vi "Tellegen's Theorem_26_08_2014.vi"() -> ()   [LabVIEW 2011]
panel:
  out "Switch 4":bool
  out "Ammeter 3":dbl(knob) scale=-5.0..5.0
  out "Switch":bool
  out "Ammeter 2":dbl(knob) scale=-5.0..5.0
  out "Switch":bool
  out "Ammeter":dbl(knob) scale=-5.0..5.0 scale format="%#.6g"
  in  "Circuit Select":enum32{"Case1 ", "Case 2", "Case 3"}(tab)
  out "Table-1(Case-1)":string[][](table)
  out "Table 2(Case-2)":string[][](table)
  out "Table 3 (case-3)":string[][](table)
  in  "Voltage(V2)":dbl
  in  "Voltage(V1)":dbl
  in  "R3":dbl=29.3001 min=1e-05 max=50.0 step=0.05
  in  "R2":dbl=119.7 min=1e-06 max=185.0 step=0.05
  in  "R1":dbl=49.8001 min=1e-05 max=85.0 step=0.05
  in  "S1(DPDT)":enum16{"POWER", "SHORT"}(ring)
  in  "S2(DPDT)":enum16{"POWER", "SHORT"}(ring)
  out "Switch 2":bool
  out "Switch 1":bool
  # "Tellegen's  Theorem"
  # "Experiment Part Select        \nSet all the resistance R1, R2, R3 and set the voltages V1 and V2.       \n   \nCase-1: Select switch of S1 and S2 . Simulate the program . Observe the result from Case 1.\n    \n Case-2: \n a) Apply switch S1 to \"Power\" and S2 to \"Short\". Simulate the program.\nObserve the all branches current  and branch volatge from Case 2 tab.\n\n \nCase-3: a) Apply switch S1 to \"Short\" and S2 to \"Power\". Simulate the program.\nObserve the all branches current  and branch volatge from Case 2 tab.\n\n\n \n    \n       MC-Moving Coil.\n       DPDT- Double pole Double throw."
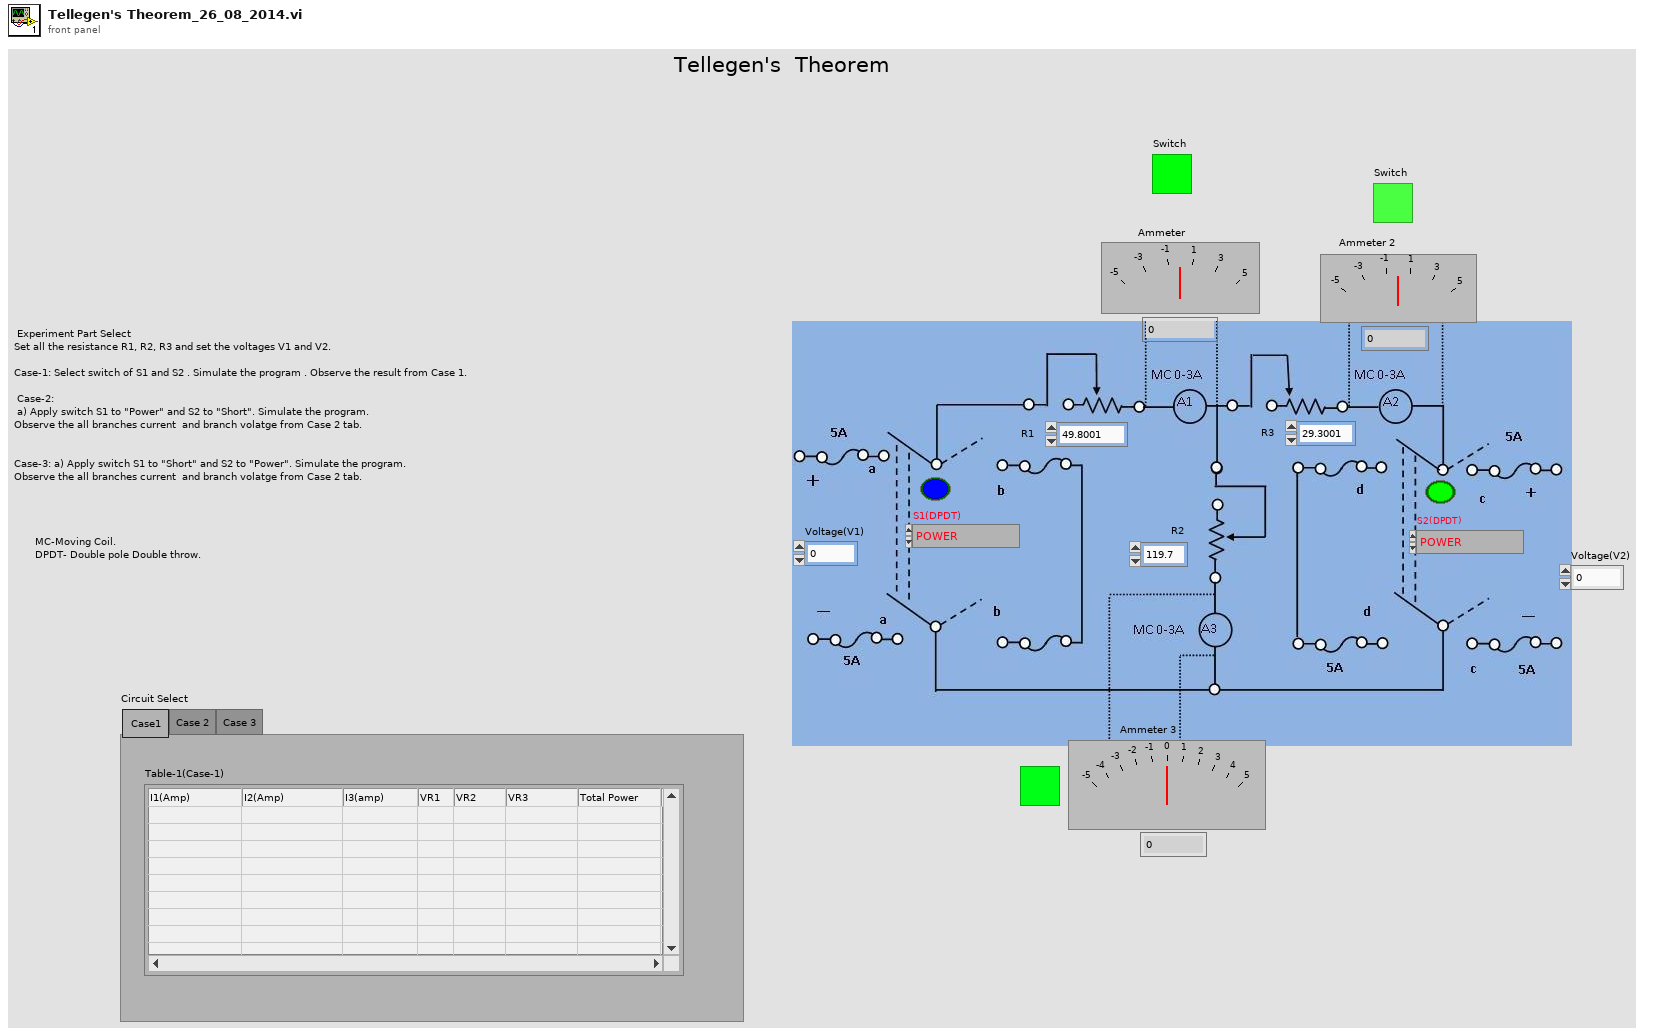
[diagram p1: front panel]
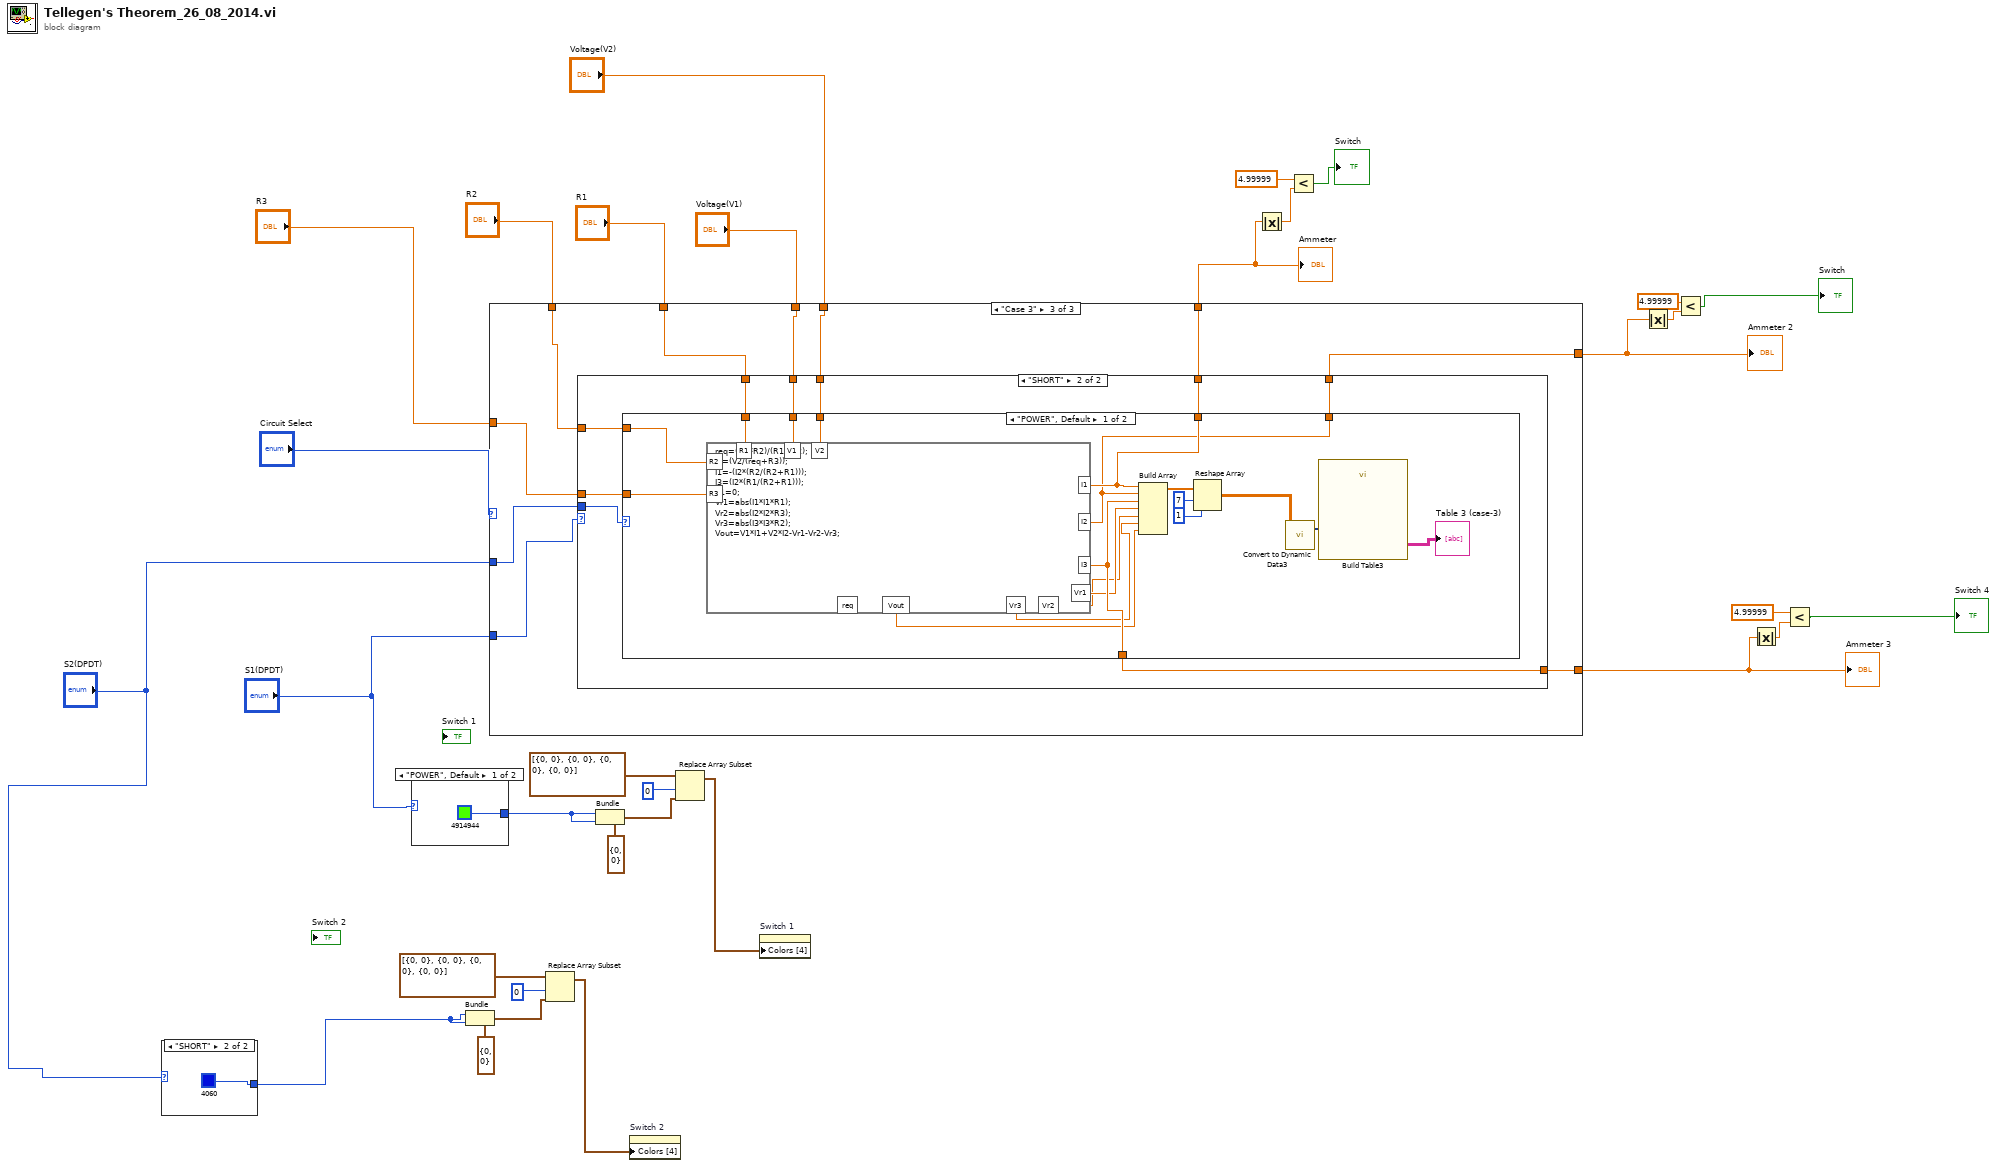
[diagram p0: block diagram]
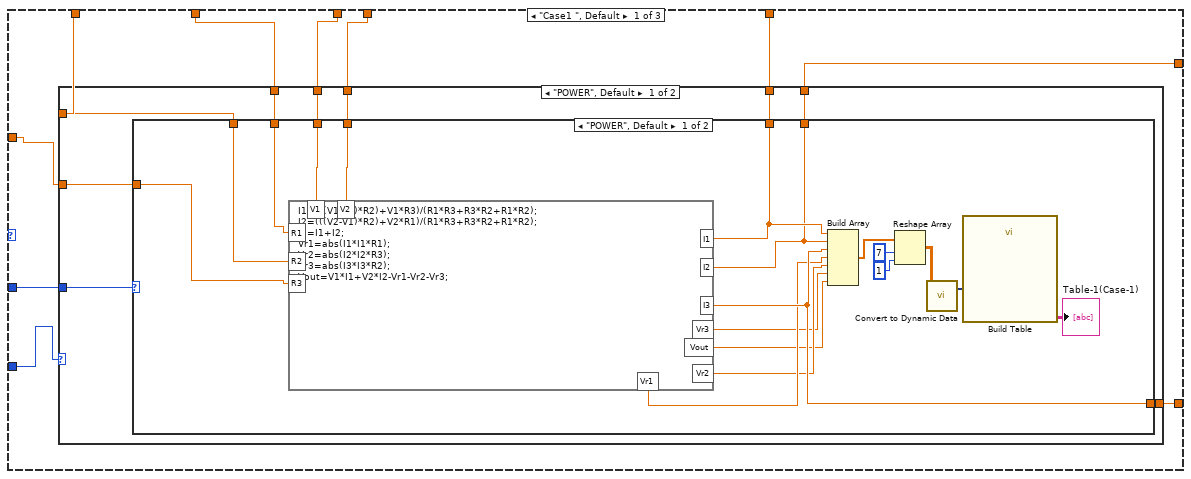
[diagram p2: hidden frame]
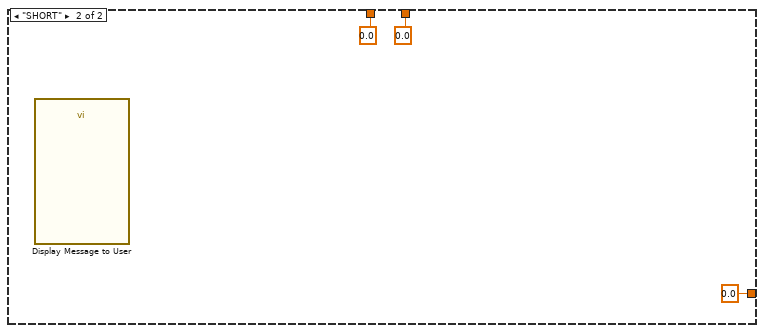
[diagram p3: hidden frame]
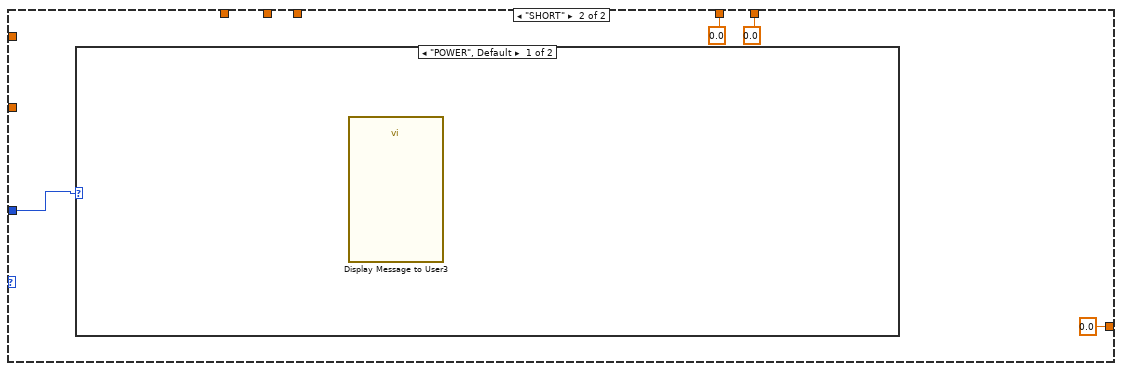
[diagram p4: hidden frame]
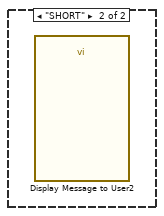
[diagram p5: hidden frame]
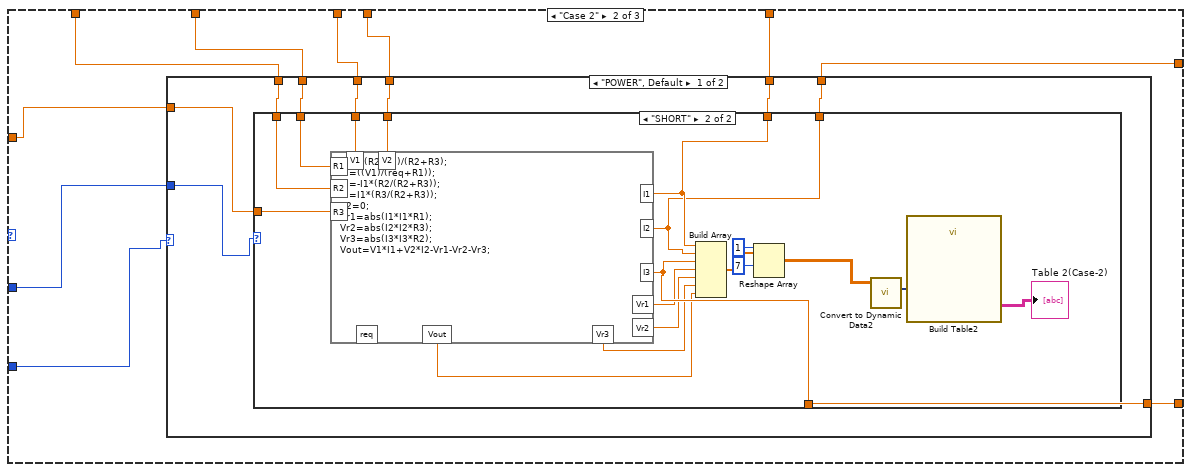
[diagram p6: hidden frame]
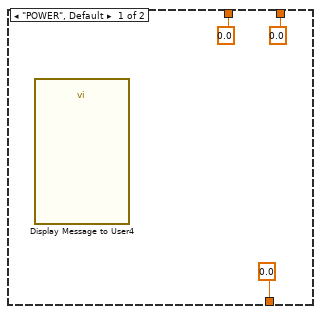
[diagram p7: hidden frame]
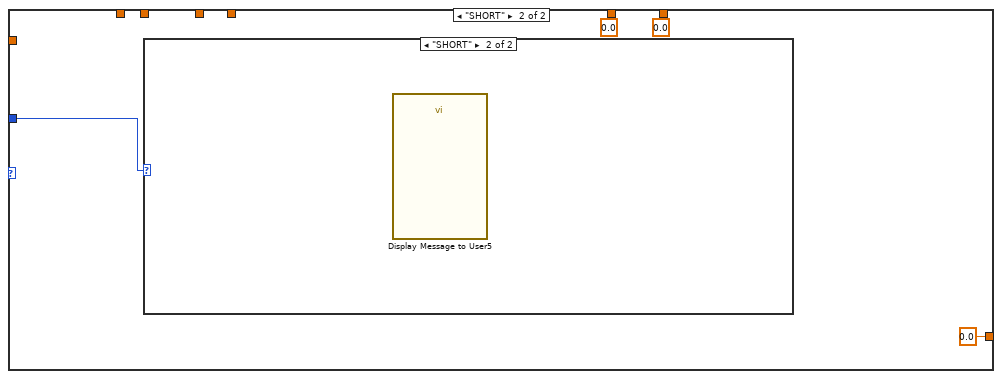
[diagram p8: hidden frame]
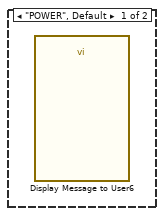
[diagram p9: hidden frame]
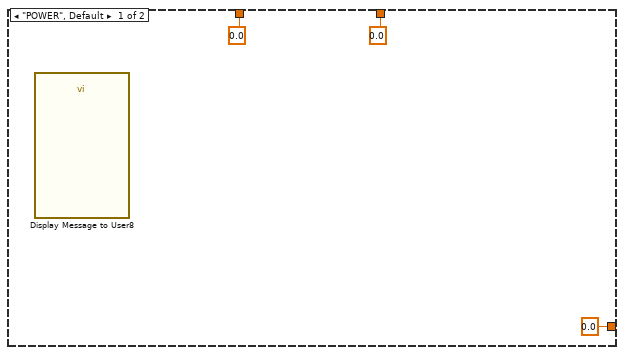
[diagram p10: hidden frame]
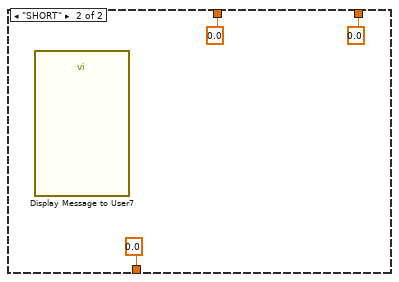
[diagram p11: hidden frame]
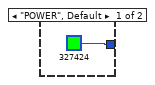
[diagram p12: hidden frame]
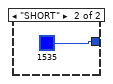
[diagram p13: hidden frame]
diagram:
  n1 = case shown="\"SHORT\"" "S2(DPDT)" {
    tunnel: [u32 327424 u32 4060] -> w21
    frame "POWER", Default {
    }
    frame "SHORT" {
    }
  }
  n2 = case shown="\"POWER\", Default" "S1(DPDT)" {
    tunnel: [u32 4914944 u32 1535] -> w28
    frame "POWER", Default {
    }
    frame "SHORT" {
    }
  }
  n3 = Bundle(cluster=cluster{u32, u32} {0, 0}, w21, w21) -> (w24:cluster{u32, u32})
  n4 = case shown="\"Case 3\"" "Circuit Select" {
    tunnel: "S1(DPDT)" -> [w41 w90 w134]
    tunnel: "Voltage(V1)" -> [w45 w87 w129]
    tunnel: "Voltage(V2)" -> [w46 w88 w128]
    tunnel: "R1" -> [w44 w86 w132]
    tunnel: "R2" -> [w43 w85 w131]
    tunnel: "R3" -> [w42 w84 w130]
    tunnel: "S2(DPDT)" -> [w40 w89 w133]
    tunnel: [w39 w83 w127] -> w9
    tunnel: [w38 w82 w126] -> w1
    tunnel: [w37 w81 w125] -> w2
    frame "Case1 ", Default {
      n5 = case shown="\"POWER\", Default" w41 {
        tunnel: w45 -> [w55 _]
        tunnel: w44 -> [w54 _]
        tunnel: w42 -> [w53 _]
        tunnel: w46 -> [w52 _]
        tunnel: w43 -> [w51 _]
        tunnel: w40 -> [w50 w80]
        tunnel: [w49 0.0 ("I1")] -> w39
        tunnel: [w48 0.0 ("I2")] -> w38
        tunnel: [w47 0.0 ("I3")] -> w37
        frame "POWER", Default {
          n6 = case shown="\"POWER\", Default" w50 {
            tunnel: w52 -> [w73 _]
            tunnel: w55 -> [w72 _]
            tunnel: w54 -> [w71 _]
            tunnel: w51 -> [w70 _]
            tunnel: w53 -> [w69 _]
            tunnel: [w62 0.0 ("I1")] -> w49
            tunnel: [w61 0.0 ("I2")] -> w48
            tunnel: [w60 0.0 ("I3")] -> w47
            frame "POWER", Default {
              n7 = formula code="I1=(((V1-V2)*R2)+V1*R3)/(R1*R3+R3*R2+R1*R2);\nI2=(((V2-V1)*R2)+V2*R1)/(R1*R3+R3*R2+R1*R2);\nI3=I1+I2;\nVr1=abs(I1*I1*R1);\nVr2=abs(I2*I2*R3);\nVr3=abs(I3*I3*R2);\nVout=V1*I1+V2*I2-Vr1-Vr2-Vr3;"("V1"=w72, "V2"=w73, "R1"=w71, "R2"=w70, "R3"=w69) -> ("I1"=w62:dbl, "I2"=w61:dbl, "I3"=w60:dbl, "Vout"=w56:dbl, "Vr1"=w59:dbl, "Vr3"=w57:dbl, "Vr2"=w58:dbl)
              n8 = Build Array(w62, w61, w60, w59, w58, w57, w56) -> (w67:dbl[])
              n9 = Reshape Array(w67, 7 ("dimension size"), 1 ("dimension size")) -> (w64:dbl[][])
              n10 = call "Convert to Dynamic Data"("2D Array"=w64) -> ("Dynamic Data Type"=w63:dynamicdata)  [unwired: 3 out]
              n11 = call "Build Table"("Signals"=w63) -> ("Table"=→"Table-1(Case-1)":string[][])  [unwired: 4 in, 6 out]
            }
            frame "SHORT" {
              n12 = call "Display Message to User"() -> ()  [unwired: 10 in, 2 out]
            }
          }
        }
        frame "SHORT" {
          n13 = case shown="\"POWER\", Default" w80 {
            frame "POWER", Default {
              n14 = call "Display Message to User3"() -> ()  [unwired: 10 in, 2 out]
            }
            frame "SHORT" {
              n15 = call "Display Message to User2"() -> ()  [unwired: 10 in, 2 out]
            }
          }
        }
      }
    }
    frame "Case 2" {
      n16 = case shown="\"POWER\", Default" w90 {
        tunnel: w89 -> [w99 w124]
        tunnel: w88 -> [w98 _]
        tunnel: w87 -> [w97 _]
        tunnel: w86 -> [w96 _]
        tunnel: w85 -> [w95 _]
        tunnel: w84 -> [w94 _]
        tunnel: [w93 0.0 ("I1")] -> w83
        tunnel: [w92 0.0 ("I2")] -> w82
        tunnel: [w91 0.0 ("I3")] -> w81
        frame "POWER", Default {
          n17 = case shown="\"SHORT\"" w99 {
            tunnel: w98 -> [_ w120]
            tunnel: w97 -> [_ w119]
            tunnel: w96 -> [_ w118]
            tunnel: w95 -> [_ w117]
            tunnel: w94 -> [_ w116]
            tunnel: [0.0 ("I1") w110] -> w93
            tunnel: [0.0 ("I2") w109] -> w92
            tunnel: [0.0 ("I3") w108] -> w91
            frame "POWER", Default {
              n18 = call "Display Message to User4"() -> ()  [unwired: 10 in, 2 out]
            }
            frame "SHORT" {
              n19 = formula code="req=(R2*R3)/(R2+R3);\nI1=((V1)/(req+R1));\nI2=-I1*(R2/(R2+R3));\nI3=I1*(R3/(R2+R3));\nV2=0;\nVr1=abs(I1*I1*R1);\nVr2=abs(I2*I2*R3);\nVr3=abs(I3*I3*R2);\nVout=V1*I1+V2*I2-Vr1-Vr2-Vr3;"("V2"=w120, "V1"=w119, "R1"=w118, "R2"=w117, "R3"=w116) -> ("I1"=w110:dbl, "I2"=w109:dbl, "I3"=w108:dbl, "Vr1"=w107:dbl, "Vr2"=w106:dbl, "Vr3"=w105:dbl, "Vout"=w103:dbl)  [unwired: 1 out]
              n20 = Build Array(w110, w109, w108, w107, w106, w105, w103) -> (w104:dbl[])
              n21 = Reshape Array(w104, 7 ("dimension size"), 1 ("dimension size")) -> (w112:dbl[][])
              n22 = call "Convert to Dynamic Data2"("2D Array"=w112) -> ("Dynamic Data Type"=w111:dynamicdata)  [unwired: 3 out]
              n23 = call "Build Table2"("Signals"=w111) -> ("Table"=→"Table 2(Case-2)":string[][])  [unwired: 4 in, 6 out]
            }
          }
        }
        frame "SHORT" {
          n24 = case shown="\"SHORT\"" w124 {
            frame "POWER", Default {
              n25 = call "Display Message to User6"() -> ()  [unwired: 10 in, 2 out]
            }
            frame "SHORT" {
              n26 = call "Display Message to User5"() -> ()  [unwired: 10 in, 2 out]
            }
          }
        }
      }
    }
    frame "Case 3" {
      n27 = case shown="\"SHORT\"" w134 {
        tunnel: w133 -> [_ w146]
        tunnel: w132 -> [_ w145]
        tunnel: w131 -> [_ w144]
        tunnel: w130 -> [_ w143]
        tunnel: w129 -> [_ w142]
        tunnel: w128 -> [_ w141]
        tunnel: [0.0 ("I1") w140] -> w127
        tunnel: [0.0 ("I2") w139] -> w126
        tunnel: [0.0 ("I3") w138] -> w125
        frame "POWER", Default {
          n28 = call "Display Message to User8"() -> ()  [unwired: 10 in, 2 out]
        }
        frame "SHORT" {
          n29 = case shown="\"POWER\", Default" w146 {
            tunnel: w145 -> [w164 _]
            tunnel: w144 -> [w163 _]
            tunnel: w143 -> [w162 _]
            tunnel: w142 -> [w161 _]
            tunnel: w141 -> [w160 _]
            tunnel: [w153 0.0 ("I1")] -> w140
            tunnel: [w152 0.0 ("I2")] -> w139
            tunnel: [w151 0.0 ("I3")] -> w138
            frame "POWER", Default {
              n30 = formula code="req=(R1*R2)/(R1+R2);\nI2=(V2/(req+R3));\nI1=-(I2*(R2/(R2+R1)));\nI3=(I2*(R1/(R2+R1)));\nV1=0;\nVr1=abs(I1*I1*R1);\nVr2=abs(I2*I2*R3);\nVr3=abs(I3*I3*R2);\nVout=V1*I1+V2*I2-Vr1-Vr2-Vr3;"("V1"=w161, "V2"=w160, "R1"=w164, "R2"=w163, "R3"=w162) -> ("I1"=w153:dbl, "I2"=w152:dbl, "I3"=w151:dbl, "Vr1"=w150:dbl, "Vr2"=w149:dbl, "Vr3"=w148:dbl, "Vout"=w147:dbl)  [unwired: 1 out]
              n31 = Build Array(w153, w152, w151, w150, w149, w148, w147) -> (w159:dbl[])
              n32 = Reshape Array(w159, 7 ("dimension size"), 1 ("dimension size")) -> (w155:dbl[][])
              n33 = call "Convert to Dynamic Data3"("2D Array"=w155) -> ("Dynamic Data Type"=w154:dynamicdata)  [unwired: 3 out]
              n34 = call "Build Table3"("Signals"=w154) -> ("Table"=→"Table 3 (case-3)":string[][])  [unwired: 4 in, 6 out]
            }
            frame "SHORT" {
              n35 = call "Display Message to User7"() -> ()  [unwired: 10 in, 2 out]
            }
          }
        }
      }
    }
  }
  "Ammeter" <- w9
  "Ammeter 2" <- w1
  "Ammeter 3" <- w2
  n36 = Replace Array Subset(array=cluster{u32, u32}[] [{0, 0}, {0, 0}, {0, 0}, {0, 0}] ("Colors [4]"), new element=w24, index=0) -> (w22:cluster{u32, u32}[])
  n37 = Bundle(cluster=cluster{u32, u32} {0, 0}, w28, w28) -> (w30:cluster{u32, u32})
  n38 = property on="Switch 2" class="Bool (strict)"("Colors [4]"=w22) -> ()  [unwired: 2 in, 2 out]
  n39 = Replace Array Subset(array=cluster{u32, u32}[] [{0, 0}, {0, 0}, {0, 0}, {0, 0}] ("Colors [4]"), new element=w30, index=0) -> (w27:cluster{u32, u32}[])
  n40 = property on="Switch 1" class="Bool (strict)"("Colors [4]"=w27) -> ()  [unwired: 2 in, 2 out]
  n41 = Absolute Value(x=w9) -> (abs(x)=w11:dbl)
  n42 = Less?(x=4.99999, y=w11) -> (x < y?=→"Switch":bool)
  n43 = Absolute Value(x=w1) -> (abs(x)=w7:dbl)
  n44 = Less?(x=4.99999, y=w7) -> (x < y?=→"Switch":bool)
  n45 = Absolute Value(x=w2) -> (abs(x)=w4:dbl)
  n46 = Less?(x=4.99999, y=w4) -> (x < y?=→"Switch 4":bool)
